vi "getData.vi"() -> (1 "Analogue Data (volts)":dbl[][](array[numeric]), 2 "Error Status":bool)   [LabVIEW 2013]
uses:
  Controls/blockTiming.ctl
  Globals/measurementGlobal.vi
panel:
  in  "display write dialog?":bool
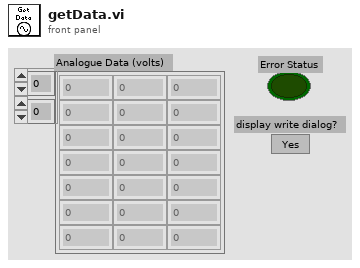
[diagram p1: front panel]
types:
  T1 = enum16{"New Measurement", "Post-process Raw Data"}
  T2 = typedef "blockTiming.ctl" = cluster{"Started":string, "Ended":string, "Analogue Frequency (Hz)":dbl}
  T3 = typedef "saveDataOption.ctl" = enum16{"Save Data", "Do Not Save Data"}
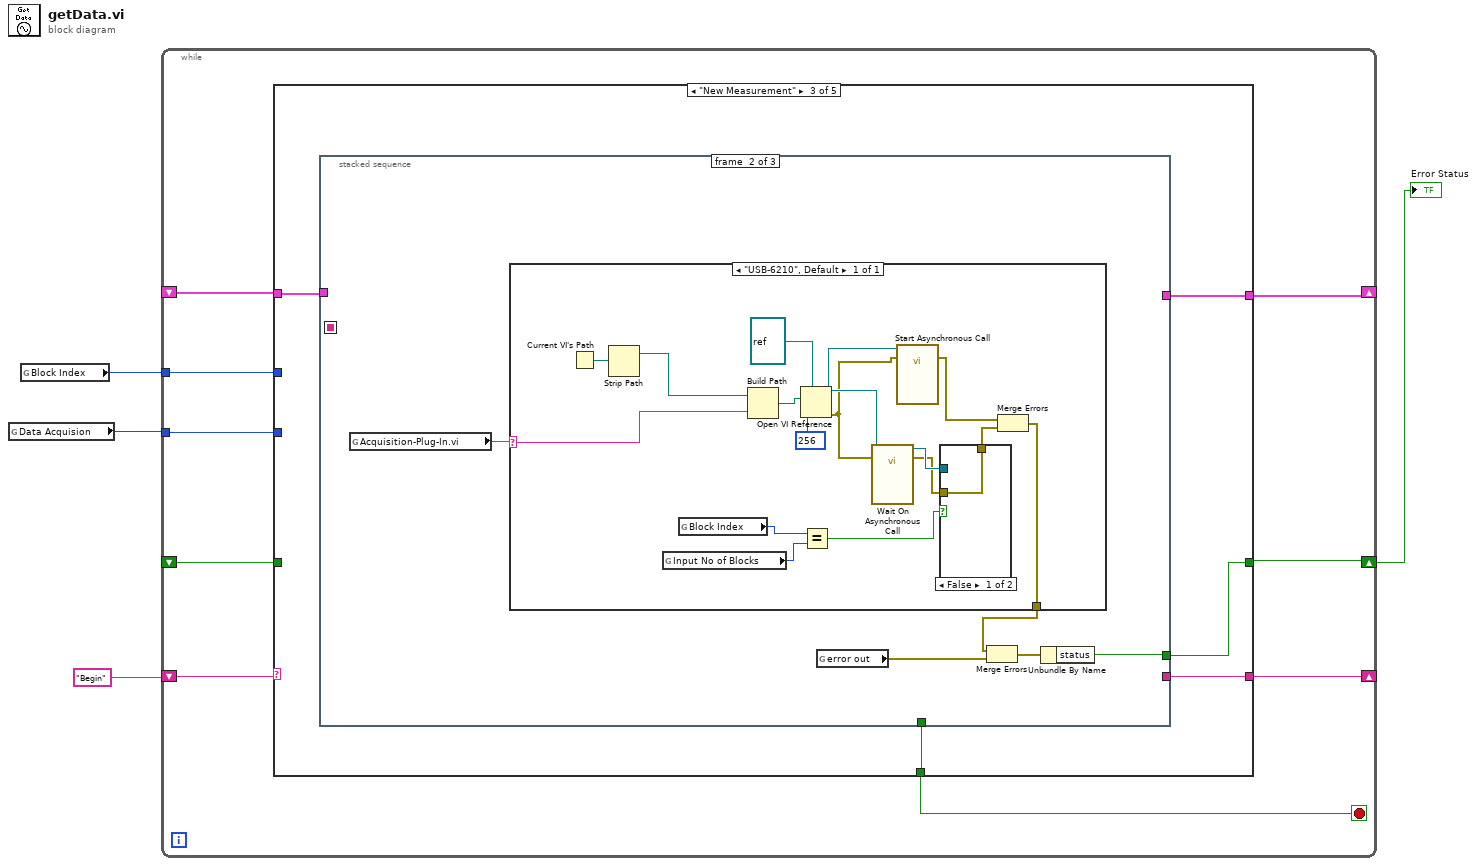
[diagram p0: block diagram]
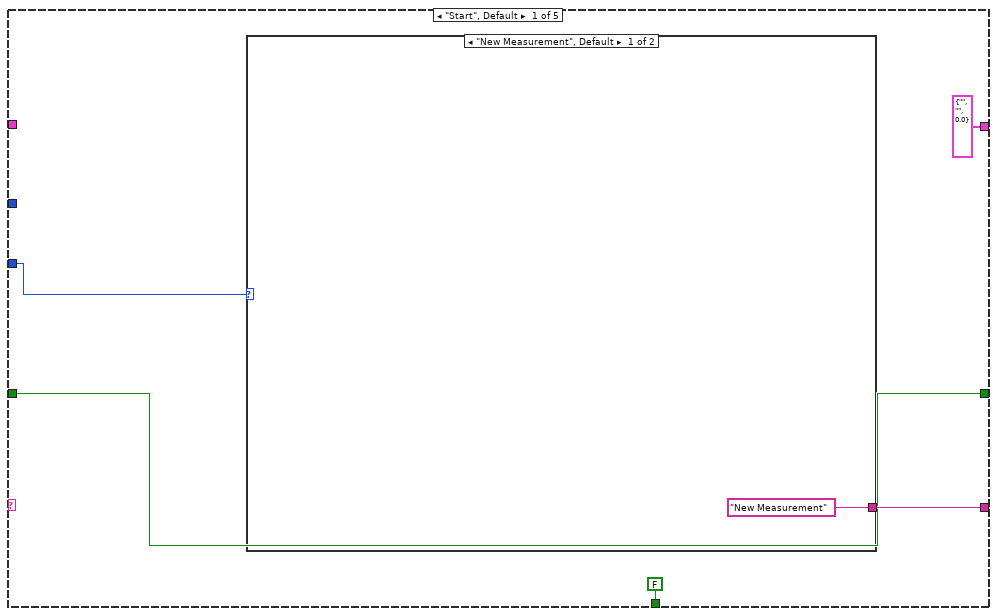
[diagram p2: hidden frame]
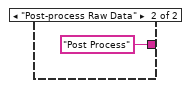
[diagram p3: hidden frame]
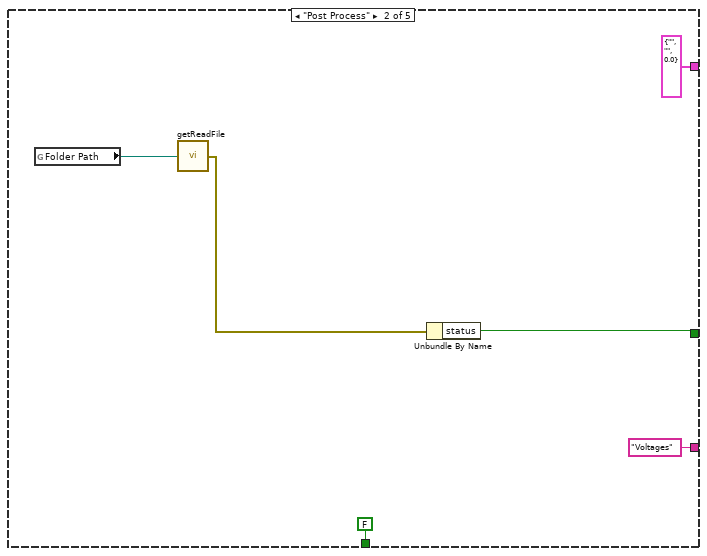
[diagram p4: hidden frame]
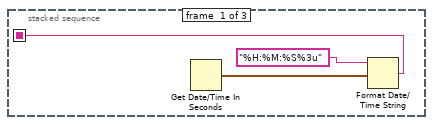
[diagram p5: hidden frame]
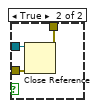
[diagram p6: hidden frame]
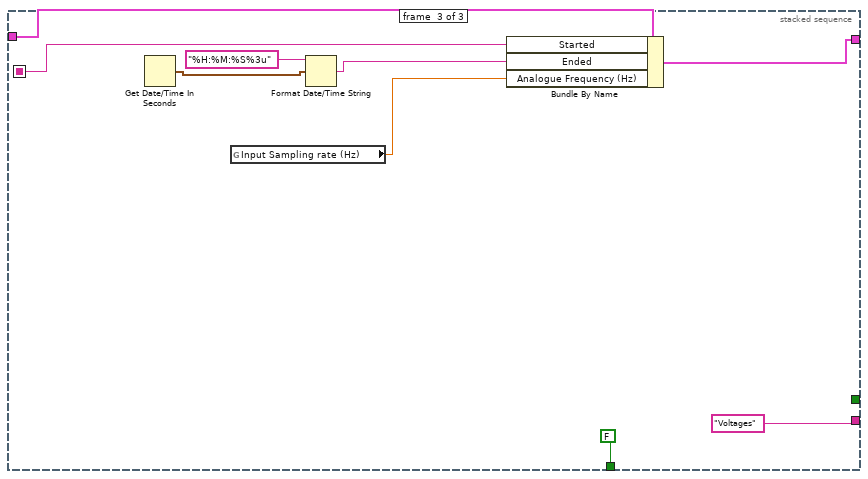
[diagram p7: hidden frame]
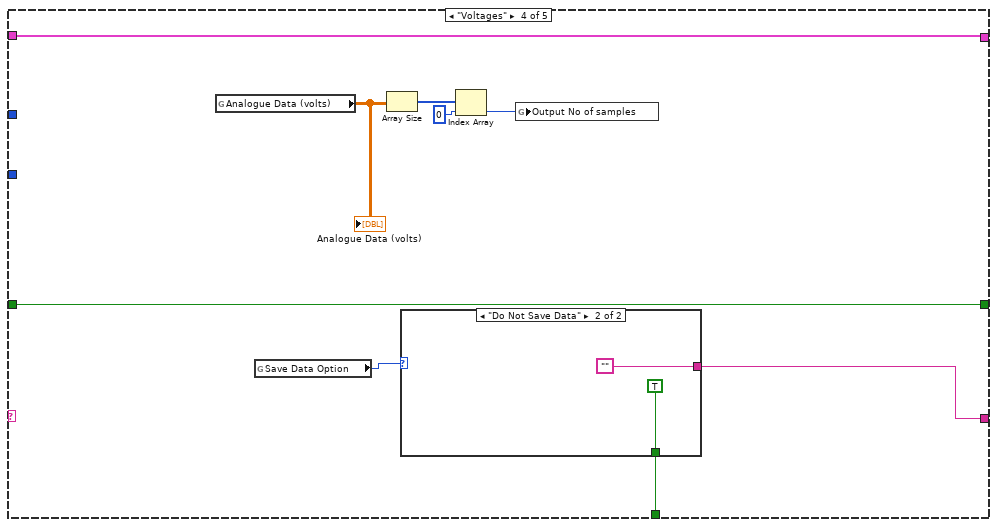
[diagram p8: hidden frame]
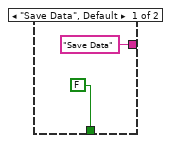
[diagram p9: hidden frame]
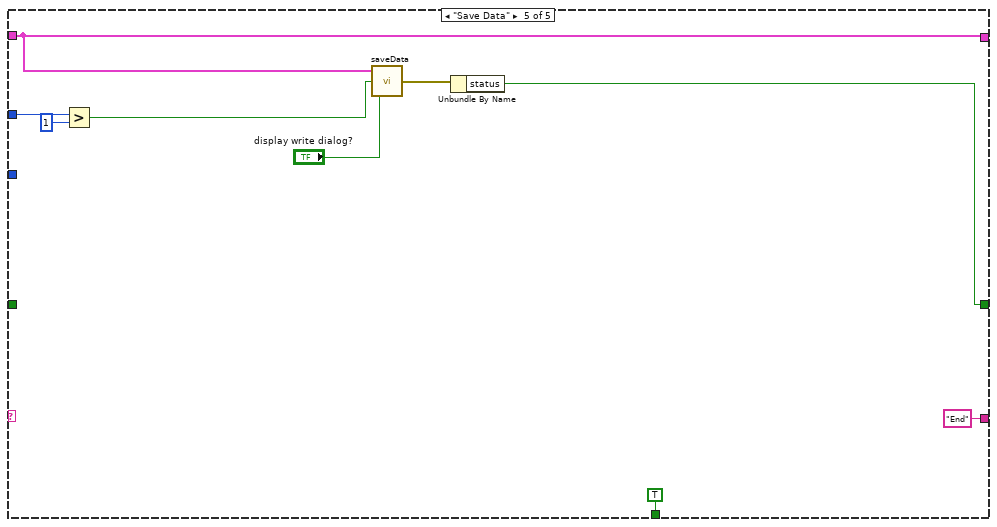
[diagram p10: hidden frame]
diagram:
  n1 = global read "measurementGlobal.vi" "Data Acquision"() -> (w3:T1)
  n2 = global read "measurementGlobal.vi" "Block Index"() -> (w1:i32)
  n3 = while {
    tunnel: w3 -> [w12]
    shift-right: [w8] -> _
    shift-left: "Begin" -> [w13]
    shift-right: [w11] -> w2
    shift-left: _ -> [w9]
    shift-right: [w6] -> _
    shift-left: _ -> [w7]
    tunnel: w1 -> [w5]
    stop <- w10 stop-if-true
    n4 = case shown="\"New Measurement\"" w13 {
      tunnel: w12 -> [w18 _ _ _ _]
      tunnel: [w17 "Voltages" w30 w70 "End"] -> w8
      tunnel: [w16 w25 w31 w72 w88] -> w11
      tunnel: [FALSE FALSE w29 w73 TRUE] -> w10
      tunnel: w9 -> [w16 _ _ w72 _]
      tunnel: w7 -> [_ _ w28 w71 w84]
      tunnel: [T2 {"Started"="", "Ended"="", "Analogue Frequency (Hz)"=0.0} ("Block Timing") T2 {"Started"="", "Ended"="", "Analogue Frequency (Hz)"=0.0} ("Block Timing") w27 w71 w84] -> w6
      tunnel: w5 -> [_ _ _ _ w90]
      frame "Start", Default {
        n5 = case shown="\"New Measurement\", Default" w18 {
          tunnel: ["New Measurement" "Post Process"] -> w17
          frame "New Measurement", Default {
          }
          frame "Post-process Raw Data" {
          }
        }
      }
      frame "Post Process" {
        n6 = global read "measurementGlobal.vi" "Folder Path"() -> (w21:path)
        n7 = call "getReadFile.vi"("Folder Path"=w21) -> ("error out"=w26:errorcluster)
        n8 = Unbundle By Name(w26) -> ("status"=w25:bool)
      }
      frame "New Measurement" {
        n9 = stacked-sequence {
          seq-local: [w33 _ _] -> [_ _ w66]
          tunnel: [_ w35 _] -> w31
          tunnel: [_ _ "Voltages"] -> w30
          tunnel: [_ _ FALSE] -> w29
          tunnel: w28 -> [_ _ w63]
          tunnel: [_ _ w64] -> w27
          frame #0 {
            n10 = Get Date/Time In Seconds() -> (seconds since 1Jan1904=w34:timestamp)
            n11 = Format Date/Time String(time format string (%c)="%H:%M:%S%3u", seconds (now)=w34) -> (date/time string=w33:string)  [unwired: 1 in]
          }
          frame #1 {
            n12 = global read "measurementGlobal.vi" "Acquisition-Plug-In.vi"() -> (w39:string)
            n13 = case shown="\"USB-6210\", Default" w39 {
              selector: w39 -> [w54]
              tunnel: [w50] -> w38
              frame "USB-6210", Default {
                n14 = Current VI's Path() -> (path=w55:path)
                n15 = Strip Path(path=w55) -> (stripped path=w43:path)  [unwired: 1 out]
                n16 = global read "measurementGlobal.vi" "Input No of Blocks"() -> (w41:i32)
                n17 = global read "measurementGlobal.vi" "Block Index"() -> (w42:i32)
                n18 = Build Path(base path=w43, name or relative path=w54) -> (appended path=w44:path)
                n19 = Open VI Reference(type specifier VI Refnum (for type only)=refnum<vi> refnum, vi path=w44, options=256) -> (vi reference=w49:refnum<vi>, error out=w48:errorcluster)  [unwired: 3 in]
                n20 = Equal?(x=w42, y=w41) -> (x = y?=w40:bool)
                n21 = call-by-ref "Wait On Asynchronous Call"(reference=w49, error in=w48) -> (reference out=w53:refnum<vi>, error out=w52:errorcluster)  [unwired: 1 in, 1 out]
                n22 = call-by-ref "Start Asynchronous Call"(reference=w49, error in=w48) -> (error out=w47:errorcluster)  [unwired: 1 in, 2 out]
                n23 = case shown="False" w40 {
                  tunnel: w53 -> [_ w59]
                  tunnel: w52 -> [w56 w58]
                  tunnel: [w56 w57] -> w51
                  frame False {
                  }
                  frame True {
                    n24 = Close Reference(reference=w59, error in (no error)=w58) -> (error out=w57:errorcluster)
                  }
                }
                n25 = Merge Errors(w47, w51) -> (w50:errorcluster)
              }
            }
            n26 = global read "measurementGlobal.vi" "error out"() -> (w37:errorcluster)
            n27 = Merge Errors(w38, w37) -> (w36:errorcluster)
            n28 = Unbundle By Name(w36) -> ("status"=w35:bool)
          }
          frame #2 {
            n29 = Get Date/Time In Seconds() -> (seconds since 1Jan1904=w61:timestamp)
            n30 = global read "measurementGlobal.vi" "Input Sampling rate (Hz)"() -> (w65:dbl)
            n31 = Format Date/Time String(time format string (%c)="%H:%M:%S%3u", seconds (now)=w61) -> (date/time string=w60:string)  [unwired: 1 in]
            n32 = Bundle By Name(cluster=w63, "Started"=w66, "Ended"=w60, "Analogue Frequency (Hz)"=w65) -> (w64:T2)
          }
        }
      }
      frame "Voltages" {
        n33 = global read "measurementGlobal.vi" "Analogue Data (volts)"() -> (w69:dbl[][])
        "Analogue Data (volts)" <- w69
        n34 = global read "measurementGlobal.vi" "Save Data Option"() -> (w74:T3)
        n35 = Array Size(array=w69) -> (size(s)=w77:i32[])
        n36 = case shown="\"Do Not Save Data\"" w74 {
          tunnel: [FALSE TRUE] -> w73
          tunnel: ["Save Data" ""] -> w70
          frame "Save Data", Default {
          }
          frame "Do Not Save Data" {
          }
        }
        n37 = Index Array(array=w77, index=0) -> (element=w75:i32)
        n38 = global write "measurementGlobal.vi" "Output No of samples"(w75) -> ()
      }
      frame "Save Data" {
        n39 = Greater?(x=w90, y=1) -> (0:w82:bool)
        n40 = call "saveData.vi"("display write dialog?"="display write dialog?", "append to file?"=w82, "Block Timing"=w84) -> ("error out"=w85:errorcluster)
        n41 = Unbundle By Name(w85) -> ("status"=w88:bool)
      }
    }
  }
  "Error Status" <- w2
